vi "set zero.vi"(11 "String in":string) -> (3 "String out":string)   [LabVIEW 2024]
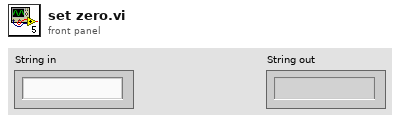
[diagram p1: front panel]
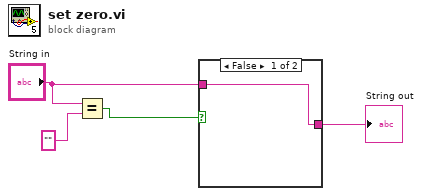
[diagram p0: block diagram]
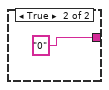
[diagram p2: hidden frame]
diagram:
  n1 = Equal?(x="String in", y="") -> (x = y?=w3:bool)
  n2 = case shown="False" w3 {
    tunnel: [w5 "0"] -> w2
    tunnel: "String in" -> [w5 _]
    frame False {
    }
    frame True {
    }
  }
  "String out" <- w2
